vi "LC_Relay_MultipleClose.vi"(6 "Reset Relay":bool, 7 "Transfer Trip":bool, 8 "Pulse Index In":i32, 9 "State In":T1(ring)=enum."Wait for Trip", 10 "Trip signal":bool, 11 "Time lapsed":u32) -> (0 "Pulse Index Out":i32, 1 "State Out":T1(ring)=enum."Wait for Trip", 2 "Reclose":bool, 3 "Lockout":bool, 4 "State":i16=-1)   [LabVIEW 2016]
doc: "Controls activation signal for reclosing VI."
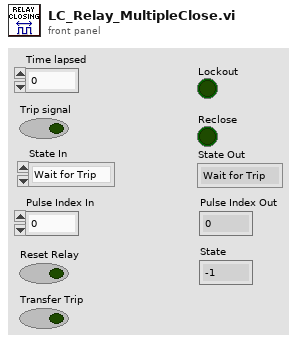
[diagram p1: front panel]
types:
  T1 = enum16{"Idle", "Wait for Trip", "PulseClosing", "Locked"}
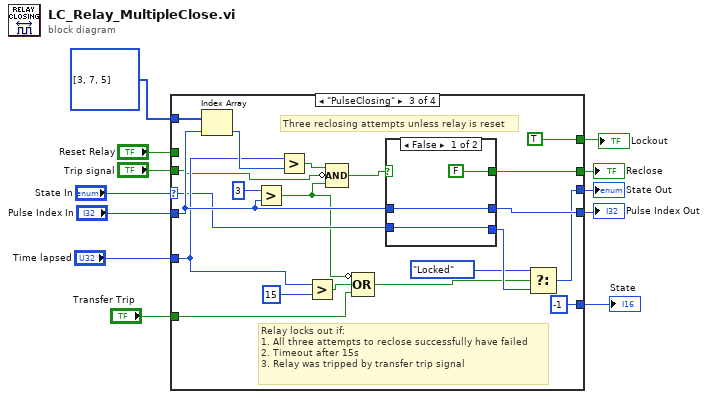
[diagram p0: block diagram]
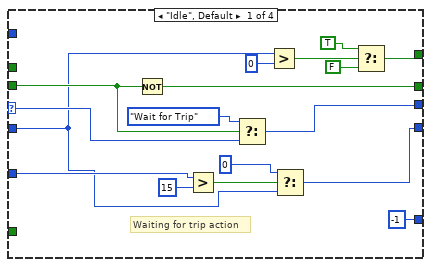
[diagram p2: hidden frame]
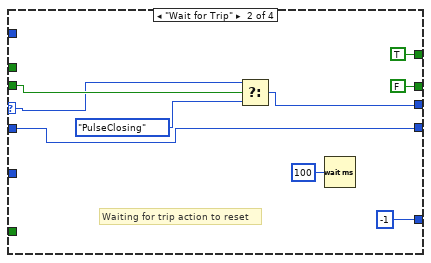
[diagram p3: hidden frame]
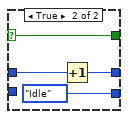
[diagram p4: hidden frame]
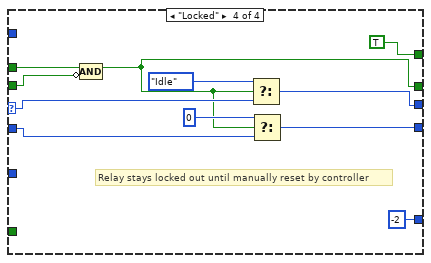
[diagram p5: hidden frame]
diagram:
  n1 = case shown="\"PulseClosing\"" "State In" {
    selector: "State In" -> [w29 w37 w46 w76]
    tunnel: [w25 FALSE w56 w70] -> w12
    tunnel: "Trip signal" -> [w26 w38 w47 w72]
    tunnel: [w27 w35 w50 w74] -> w4
    tunnel: "Pulse Index In" -> [w15 w33 w53 w77]
    tunnel: "Reset Relay" -> [_ _ _ w73]
    tunnel: u32[] [3, 7, 5] -> [_ _ w55 _]
    tunnel: [w14 w33 w54 w71] -> w7
    tunnel: "Time lapsed" -> [w16 _ w51 _]
    tunnel: [w24 TRUE ("Lockout") TRUE ("Lockout") TRUE ("Lockout")] -> w3
    tunnel: "Transfer Trip" -> [_ _ w40 _]
    tunnel: [i16 -1 ("Numeric") i16 -1 ("Numeric") i16 -1 ("Numeric") i16 -2 ("Numeric")] -> w1
    frame "Idle", Default {
      # "Waiting for trip action"
      n2 = Not(x=w26) -> (.not. x?=w25:bool)
      n3 = Greater?(x=w16, y=u32 15) -> (0:w17:bool)
      n4 = Select(t=T1."Wait for Trip", s=w26, f=w29) -> (s? t:f=w27:T1)
      n5 = Greater?(x=w15, y=0) -> (0:w21:bool)
      n6 = Select(t=0 ("y"), s=w17, f=w15) -> (s? t:f=w14:i32)
      n7 = Select(t=TRUE ("Lockout"), s=w21, f=FALSE) -> (s? t:f=w24:bool)
    }
    frame "Wait for Trip" {
      # "Waiting for trip action to reset"
      n8 = Select(t=w37, s=w38, f=T1."PulseClosing") -> (s? t:f=w35:T1)
      n9 = Wait (ms)(milliseconds to wait=u32 100) -> ()  [unwired: 1 out]
    }
    frame "PulseClosing" {
      # "Relay locks out if:\n1. All three attempts to reclose successfully have failed\n2. Timeout after 15s\n3. Relay was tripped by transfer trip signal"
      # "Three reclosing attempts unless relay is reset"
      n10 = Index Array(array=w55, index=w53) -> (element=w52:u32)
      n11 = Greater?(x=3, y=w53) -> (0:w44:bool)
      n12 = Greater?(x=w51, y=w52) -> (0:w58:bool)
      n13 = Greater?(x=w51, y=u32 15) -> (0:w48:bool)
      n14 = Compound Arithmetic op=AND(w58, invert w47, w44) -> (w57:bool)
      n15 = Compound Arithmetic op=OR(invert w44, w48, w40) -> (w43:bool)
      n16 = case shown="False" w57 {
        selector: w57 -> [_ w66]
        tunnel: [FALSE w66] -> w56
        tunnel: [w61 w65] -> w54
        tunnel: w53 -> [w61 w64]
        tunnel: [w60 T1."Idle"] -> w45
        tunnel: w46 -> [w60 _]
        frame False {
        }
        frame True {
          n17 = Increment(x=w64) -> (x+1=w65:i32)
        }
      }
      n18 = Select(t=T1."Locked", s=w43, f=w45) -> (s? t:f=w50:T1)
    }
    frame "Locked" {
      # "Relay stays locked out until manually reset by controller"
      n19 = Compound Arithmetic op=AND(w73, invert w72) -> (w70:bool)
      n20 = Select(t=T1."Idle", s=w70, f=w76) -> (s? t:f=w74:T1)
      n21 = Select(t=0 ("Pulse Index In"), s=w70, f=w77) -> (s? t:f=w71:i32)
    }
  }
  "Reclose" <- w12
  "Pulse Index Out" <- w7
  "State Out" <- w4
  "Lockout" <- w3
  "State" <- w1
